vi "LVFunction_Get installed Camera list.vi"(11 "error in (no error)":errorcluster) -> (4 "Array_Of_HASO_specifications":T1[](array[typedef]), 6 "ArrayOfConfigFilePath":path[](array[path]), 8 "Installed sensors":string[](array[string]))   [LabVIEW 2020]
uses:
  CameraSpecifications.ctl
  General dimensions definition.ctl
  Point2D.ctl
  Point2Df.ctl
  Data alignment enum.ctl
panel:
  in  "String 2":string
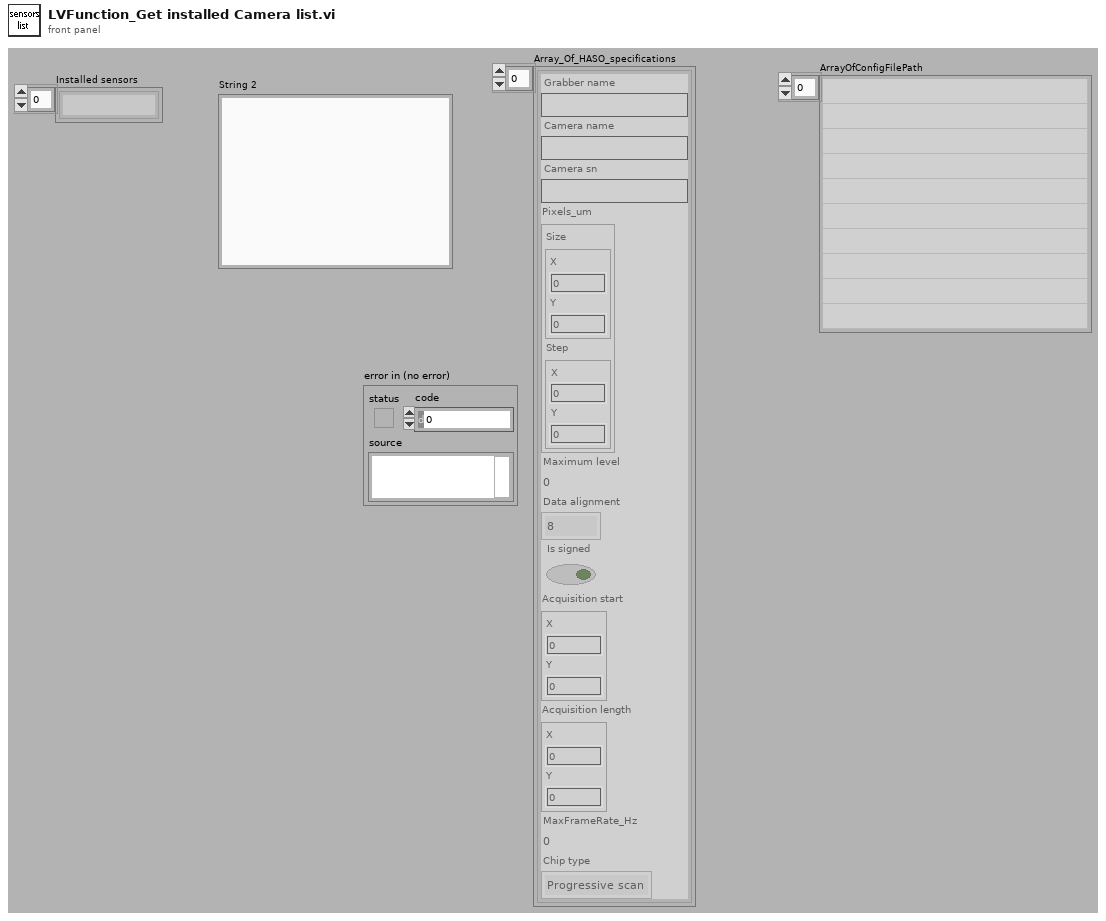
[diagram p1: front panel]
types:
  T1 = typedef "CameraSpecifications.ctl" = cluster{"Grabber name":string, "Camera name":string, "Camera sn":string, "Pixels_um":T2, "Maximum level":u32, "Data alignment":T5, "Is signed":bool, "Acquisition start":T3, "Acquisition length":T3, "MaxFrameRate_Hz":sgl, "Chip type":enum16{"Progressive scan", "Frame transfert"}}
  T2 = typedef "General dimensions definition.ctl" = cluster{"Size":T3, "Step":T4}
  T3 = typedef "Point2D.ctl" = cluster{"X":u32, "Y":u32}
  T4 = typedef "Point2Df.ctl" = cluster{"X":sgl, "Y":sgl}
  T5 = typedef "Data alignment enum.ctl" = enum16{"8", "16", "32"}
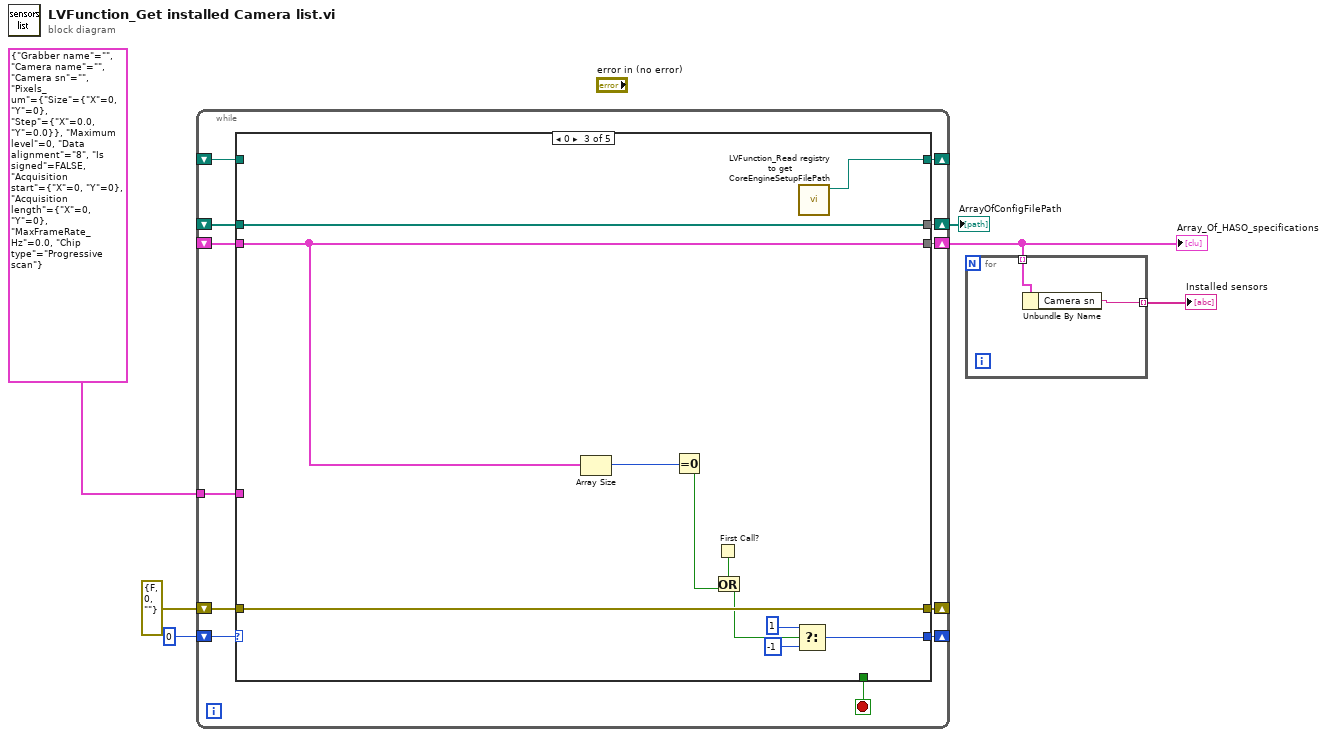
[diagram p0: block diagram]
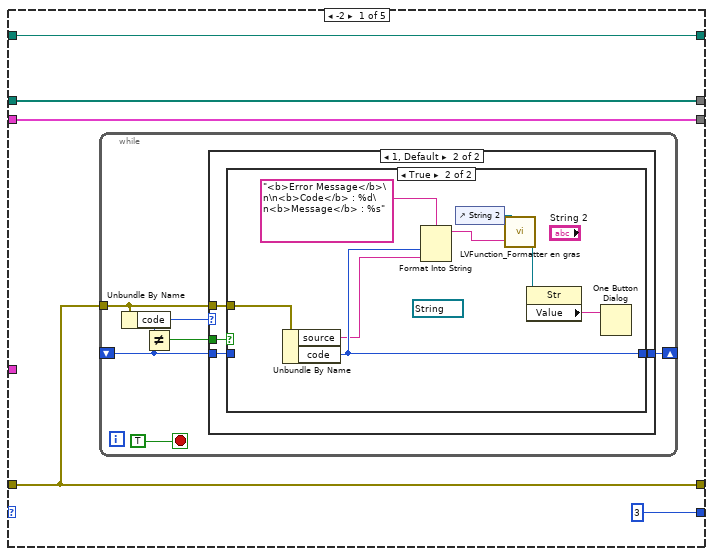
[diagram p2: hidden frame]
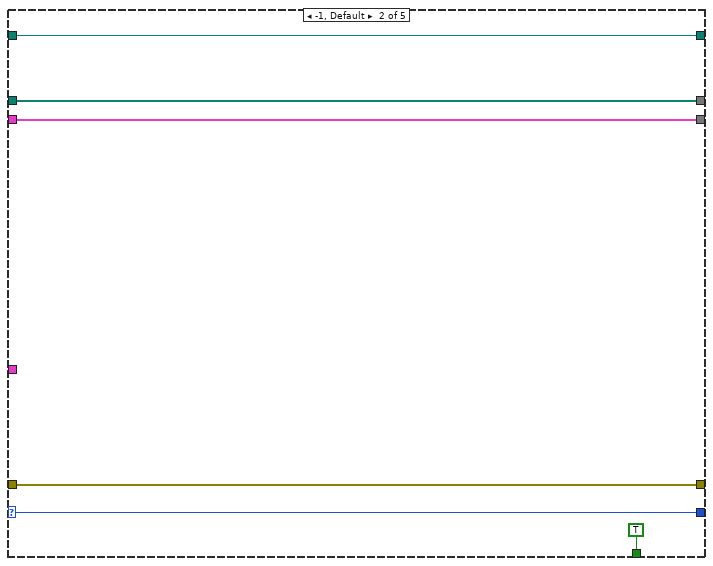
[diagram p5: hidden frame]
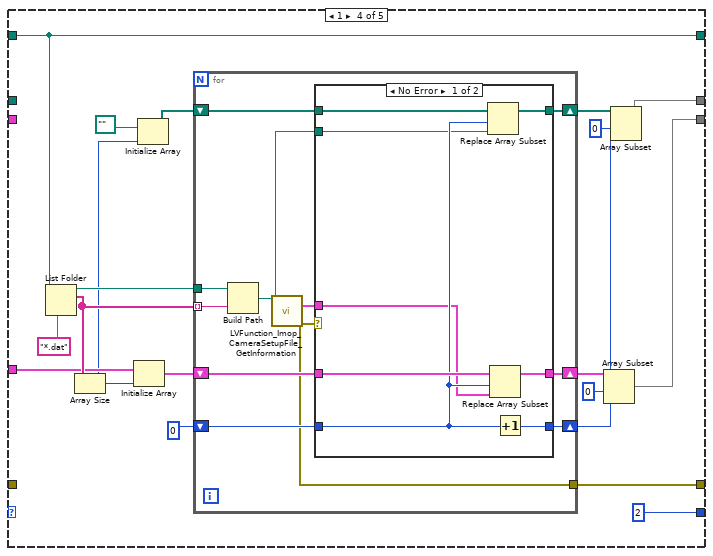
[diagram p6: hidden frame]
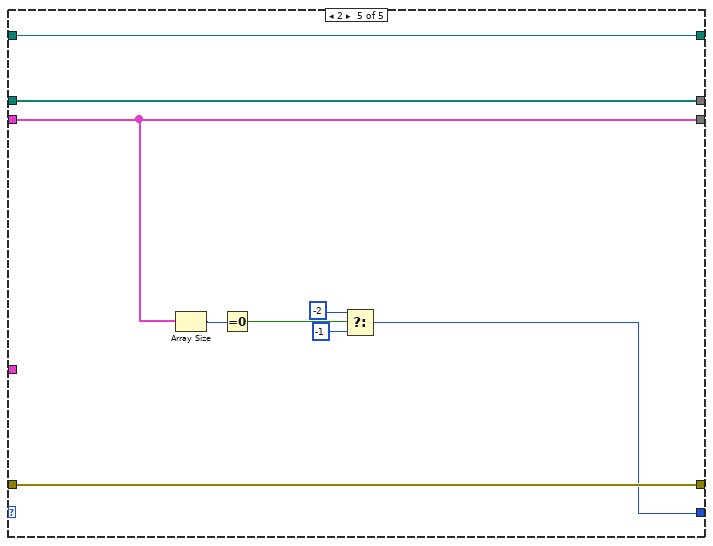
[diagram p8: hidden frame]
diagram:
  n1 = while {
    shift-right: [w13] -> _
    shift-left: 0 -> [w18]
    shift-right: [w16] -> w4
    shift-left: _ -> [w15]
    tunnel: T1 {"Grabber name"="", "Camera name"="", "Camera sn"="", "Pixels_um"={"Size"={"X"=0, "Y"=0}, "Step"={"X"=0.0, "Y"=0.0}}, "Maximum level"=0, "Data alignment"=enum."8", "Is signed"=FALSE, "Acquisition start"={"X"=0, "Y"=0}, "Acquisition length"={"X"=0, "Y"=0}, "MaxFrameRate_Hz"=0.0, "Chip type"=enum."Progressive scan"} ("Camera Config") -> [w17]
    shift-right: [w11] -> _
    shift-left: errorcluster {"status"=FALSE, "code"=0, "source"=""} ("error out") -> [w12]
    shift-right: [w10] -> w2
    shift-left: _ -> [w9]
    shift-right: [w8] -> _
    shift-left: _ -> [w7]
    stop <- w14 stop-if-true
    n2 = case shown="0" w18 {
      selector: w18 -> [_ w47 _ _ _]
      tunnel: w17 -> [_ _ _ w76 _]
      tunnel: [w21 w49 w58 w72 w102] -> w16
      tunnel: w15 -> [w21 w49 w58 _ w102]
      tunnel: [_ TRUE _ _ _] -> w14
      tunnel: [3 w47 w54 2 w105] -> w13
      tunnel: w12 -> [w23 w46 w60 _ w110]
      tunnel: [w23 w46 w60 w69 w110] -> w11
      tunnel: [w20 w45 w59 w64 w109] -> w10
      tunnel: w9 -> [w20 w45 w59 _ w109]
      tunnel: [w19 w44 w50 w62 w108] -> w8
      tunnel: w7 -> [w19 w44 _ w62 w108]
      frame -2 {
        n3 = while {
          tunnel: w23 -> [w29]
          shift-right: [w28] -> _
          shift-left: _ -> [w27]
          stop <- TRUE stop-if-true
          n4 = Unbundle By Name(w29) -> ("code"=w24:i32)
          n5 = Not Equal?(x=w24, y=w27) -> (x != y?=w25:bool)
          n6 = case shown="1, Default" w24 {
            selector: w24 -> [w30 _]
            tunnel: w29 -> [_ w34]
            tunnel: [w30 w33] -> w28
            tunnel: w27 -> [_ w32]
            tunnel: w25 -> [_ w31]
            frame 0 {
            }
            frame 1, Default {
              n7 = case shown="True" w31 {
                tunnel: w34 -> [_ w43]
                tunnel: [w35 w42] -> w33
                tunnel: w32 -> [w35 _]
                frame False {
                }
                frame True {
                  (unwired) refnum<vi> refnum ("String to Format (not a refnum)")
                  n8 = Unbundle By Name(w43) -> ("source"=w41:string, "code"=w42:i32)
                  n9 = Format Into String(format string="<b>Error Message</b>\n\n<b>Code</b> : %d\n<b>Message</b> : %s" ("initial string"), w42, w41) -> (resulting string=w37:string)  [unwired: 2 in, 1 out]
                  n10 = control-ref of="String 2"() -> (w38:refnum<vi>)
                  n11 = call "LVFunction_Formatter en gras.vi"("Chaîne"=w37, "Contrôle chaîne"=w38) -> ("Contrôle chaîne (dup)"=w36:refnum<vi>)  [unwired: 1 in]
                  n12 = property class="Str"(reference=w36) -> ("Value"=w39:string)  [unwired: 1 in, 2 out]
                  n13 = One Button Dialog(message=w39) -> ()  [unwired: 1 in, 1 out]
                }
              }
            }
          }
        }
      }
      frame -1, Default {
      }
      frame 0 {
        n14 = Array Size(array=w58) -> (size(s)=w57:i32)
        n15 = Equal To 0?(x=w57) -> (x = 0?=w52:bool)
        n16 = First Call?() -> (First Call?: T/F=w53:bool)
        n17 = Or(x=w53, y=w52) -> (x .or. y?=w51:bool)
        n18 = Select(t=1, s=w51, f=-1) -> (s? t:f=w54:i32)
        n19 = call "LVFunction_Read registry to get CoreEngineSetupFilePath.vi"() -> ("Path to config files"=w50:path)  [unwired: 6 in, 1 out]
      }
      frame 1 {
        n20 = List Folder(path=w62, pattern="*.dat") -> (path out=w78:path, filenames=w77:string[])  [unwired: 2 in, 2 out]
        n21 = Array Size(array=w77) -> (size(s)=w68:i32)
        n22 = Initialize Array(w76, w68) -> (w75:T1[])
        n23 = Initialize Array(path "" ("appended path"), w68) -> (w63:path[])
        n24 = for {
          tunnel: w78 -> [w90]
          tunnel: w77 -> [w89] mode=indexing
          shift-right: [w86] -> w73
          shift-left: w75 -> [w88]
          shift-right: [w84] -> w61
          shift-left: 0 -> [w87]
          tunnel: [w83] -> w69
          shift-right: [w81] -> w65
          shift-left: w63 -> [w82]
          n25 = Build Path(base path=w90, name or relative path=w89) -> (appended path=w80:path)
          n26 = call "LVFunction_Imop_CameraSetupFile_GetInformation.vi"("module path"=w80) -> ("Camera Config"=w85:T1, "error out"=w83:errorcluster)  [unwired: 13 in]
          n27 = case shown="No Error" w83 {
            tunnel: w88 -> [w98 w101]
            tunnel: w87 -> [w93 w100]
            tunnel: [w97 w101] -> w86
            tunnel: w85 -> [w91 _]
            tunnel: [w96 w100] -> w84
            tunnel: w82 -> [w95 w99]
            tunnel: [w94 w99] -> w81
            tunnel: w80 -> [w92 _]
            frame No Error {
              n28 = Replace Array Subset(array=w95, new element=w92, index=w93) -> (w94:path[])
              n29 = Replace Array Subset(array=w98, new element=w91, index=w93) -> (w97:T1[])
              n30 = Increment(x=w93) -> (x+1=w96:i32)
            }
            frame Error {
            }
          }
        }
        n31 = Array Subset(array=w73, index=0, length=w61) -> (w72:T1[])
        n32 = Array Subset(array=w65, index=0, length=w61) -> (w64:path[])
      }
      frame 2 {
        n33 = Array Size(array=w102) -> (size(s)=w107:i32)
        n34 = Equal To 0?(x=w107) -> (x = 0?=w106:bool)
        n35 = Select(t=-2, s=w106, f=-1) -> (s? t:f=w105:i32)
      }
    }
  }
  "Array_Of_HASO_specifications" <- w4
  "ArrayOfConfigFilePath" <- w2
  n36 = for {
    tunnel: w4 -> [w112] mode=indexing
    tunnel: [w111] -> w3 mode=indexing
    n37 = Unbundle By Name(w112) -> ("Camera sn"=w111:string)
  }
  "Installed sensors" <- w3
